vi "Global 1.vi"() -> ()   [LabVIEW 2017]
panel:
  out "Background":dbl
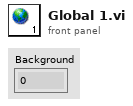
[diagram p1: front panel]
diagram:
